vi "correction_data.vi"() -> ()   [LabVIEW 2020]
uses:
  CasaoManagerGeneralSpecifications.ctl
  General dimensions definition.ctl
  Point2D.ctl
  Point2Df.ctl
  Camera.lvclass
  WavefrontCorrector.lvclass
  CorrectionDataManager.lvclass
  Image.lvclass
  HasoEngine.lvclass
  InteractionMatrixToCommandMatrixParameters.ctl
  InteractionMatrixAcquisitionParameters.ctl
  HasoSlopes.lvclass
panel:
  in  "init_state_from_config_file":bool
  out "Camera Image (command 2)":u32[][](graph)
  in  "Start Acq":bool
  out "Singular values":dbl[](graph)
  in  "Correction data file name":string="Data\\data_correction_manager_example.aoc"
  in  "Exposure time (us)":i32=1000 min=1
  in  "number of images to sum":u32=1 min=1
  out "Camera Image (command 1)":u32[][](graph)
  in  "WavefrontCorrector Configuration file path":path
  out "error out":errorcluster
  out "Informations extracted \nfrom configuration files":T1 caption="Informations extracted from configuration files"
  in  "Haso configuration file path":path
  # "This example is Hardware-dependant, \nplease use your own Haso and corrector configuration file and acquisition system"
  # "Acquisition parameters"
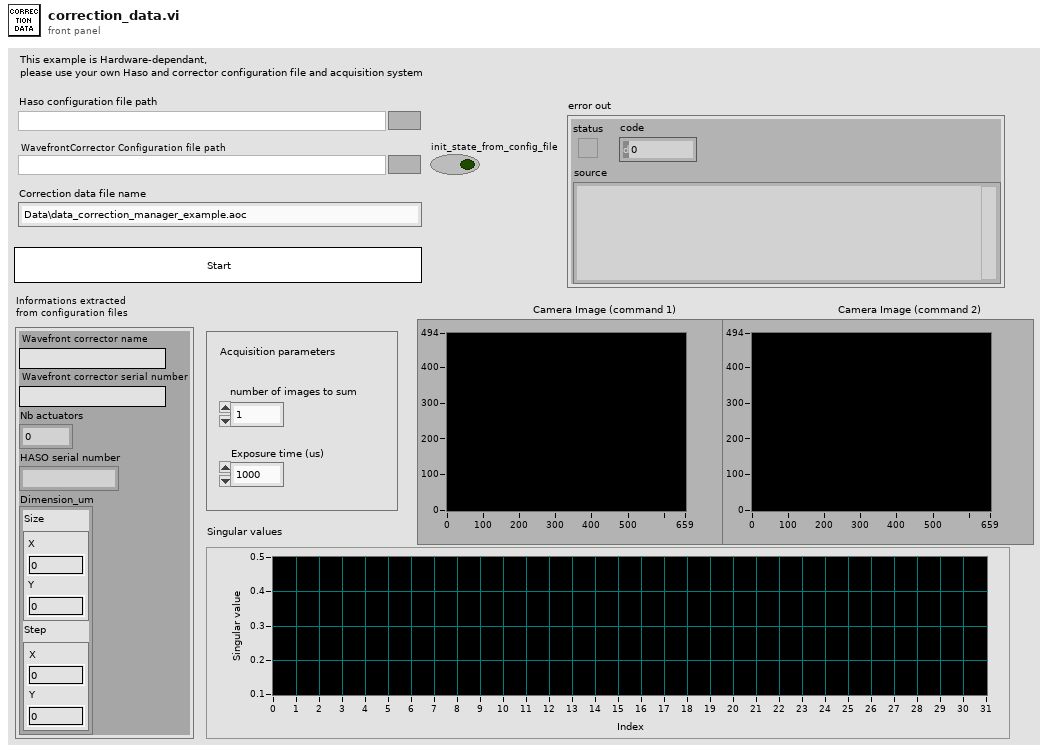
[diagram p1: front panel]
types:
  T1 = typedef "CasaoManagerGeneralSpecifications.ctl" = cluster{"Wavefront corrector name":string, "Wavefront corrector serial number":string, "Nb actuators":i32, "HASO serial number":string, "Dimension_um":T2}
  T2 = typedef "General dimensions definition.ctl" = cluster{"Size":T3, "Step":T4}
  T3 = typedef "Point2D.ctl" = cluster{"X":u32, "Y":u32}
  T4 = typedef "Point2Df.ctl" = cluster{"X":sgl, "Y":sgl}
  T5 = typedef "InteractionMatrixAcquisitionParameters.ctl" = cluster{"Push - Pull value":sgl}
  T6 = typedef "InteractionMatrixToCommandMatrixParameters.ctl" = cluster{"Number of kept modes":i32, "Tilt filtering":bool}
  T7 = typedef "Data alignment enum.ctl" = enum16{"8", "16", "32"}
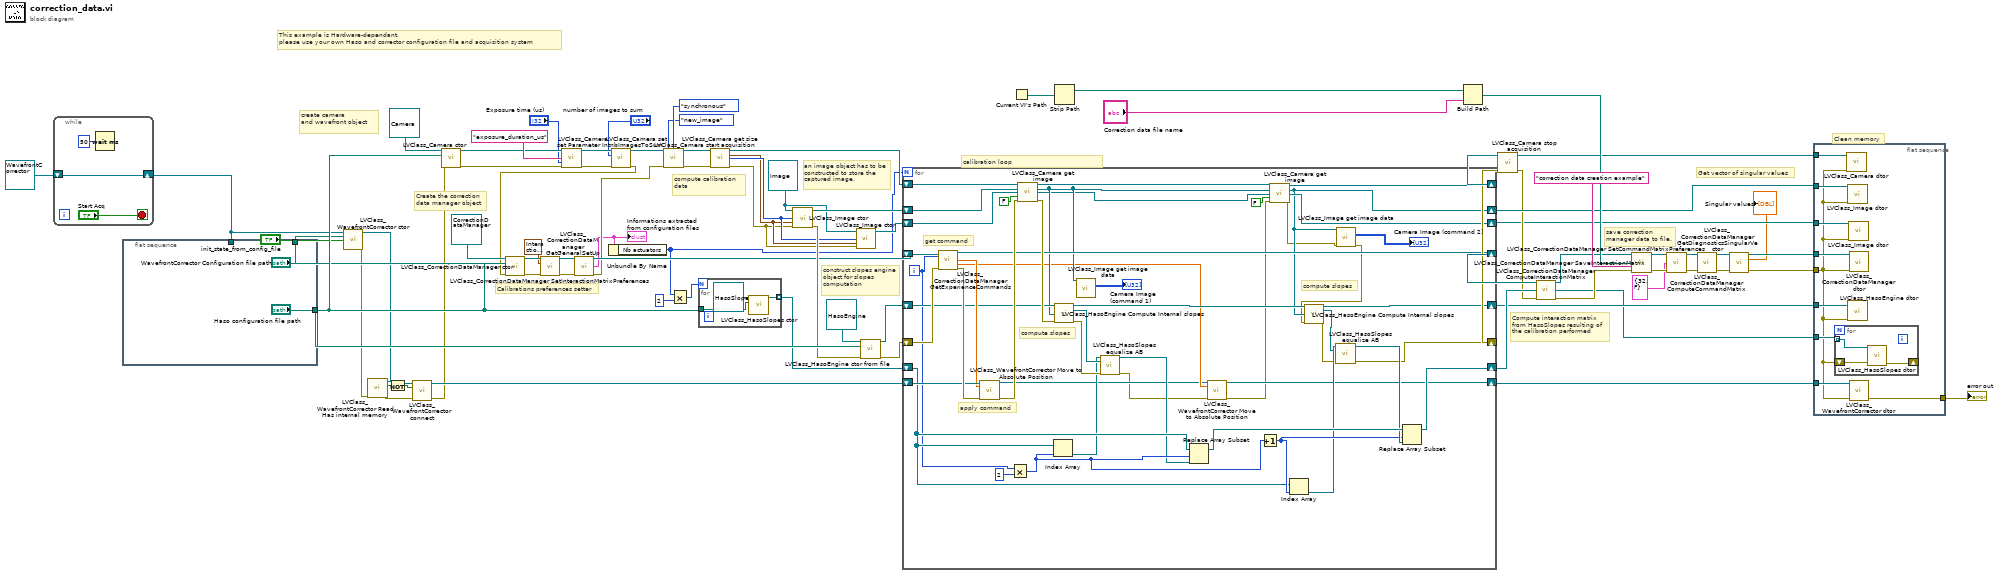
[diagram p0: block diagram]
diagram:
  w40 = refnum<class "Image.lvclass"> refnum ("Image in")
  # "Clean memory"
  # "Get vector of singular values"
  # "save correction\nmanager data to file."
  # "Compute interaction matrix\nfrom HasoSlopes resulting of\nthe calibration performed"
  # "calibration loop"
  # "construct slopes engine object for slopes computation"
  # "an image object has to be\nconstructed to store the\ncaptured image."
  # "compute calibration\ndata"
  # "Calibrations preferences setter"
  # "Create the correction\ndata manager object"
  # "create camera \nand wavefront object"
  # "This example is Hardware-dependant, \nplease use your own Haso and corrector configuration file and acquisition system"
  n1 = while {
    shift-right: [w82] -> w17
    shift-left: refnum<class "WavefrontCorrector.lvclass"> refnum ("WavefrontCorrector in") -> [w82]
    stop <- "Start Acq" stop-if-true
    n2 = Wait (ms)(milliseconds to wait=u32 50) -> ()  [unwired: 1 out]
  }
  n3 = flat-sequence {
    tunnel: ["Haso configuration file path"] -> w80
    tunnel: ["WavefrontCorrector Configuration file path"] -> w79
    tunnel: w17 -> [_]
    frame #0 {
    }
  }
  n4 = call "LVClass_WavefrontCorrector ctor.vi"("WavefrontCorrector (const)"=w17, "PathToWavefrontCorrectorSetupFile"=w79, "init_state_from_config_file"="init_state_from_config_file") -> ("WavefrontCorrector (new)"=w5:refnum<class "WavefrontCorrector.lvclass">, "error out"=w4:errorcluster)  [unwired: 11 in]
  n5 = call "LVClass_WavefrontCorrector Read Has internal memory.vi"("error in (no error)"=w4, "WavefrontCorrector in"=w5) -> ("error out"=w3:errorcluster, "Has internal memory ?"=w13:bool, "WavefrontCorrector out"=w14:refnum<class "WavefrontCorrector.lvclass">)  [unwired: 7 in]
  n6 = Not(x=w13) -> (.not. x?=w12:bool)
  n7 = call "LVClass_WavefrontCorrector connect.vi"("WavefrontCorrector in"=w14, "set_init_state_from_config_file"=w12, "error in (no error)"=w3) -> ("WavefrontCorrector out"=w15:refnum<class "WavefrontCorrector.lvclass">, "error out"=w2:errorcluster)  [unwired: 11 in]
  n8 = call "LVClass_Camera ctor.vi"("Camera (const)"=refnum<class "Camera.lvclass"> refnum ("Camera"), "Configuration file path"=w80, "error in (no error)"=w2) -> ("Camera (new)"=w28:refnum<class "Camera.lvclass">, "error out"=w22:errorcluster)  [unwired: 11 in]
  n9 = call "LVClass_Camera set Parameter Int.vi"("Camera in"=w28, "parameter_name"="exposure_duration_us", "value"="Exposure time (us)", "error in (no error)"=w22) -> ("Camera out"=w26:refnum<class "Camera.lvclass">, "error out"=w21:errorcluster)  [unwired: 10 in]
  n10 = call "LVClass_Camera set nbImagesToSum.vi"("Camera in"=w26, "nb_image"="number of images to sum", "error in (no error)"=w21) -> ("Camera out"=w25:refnum<class "Camera.lvclass">, "error out"=w20:errorcluster)  [unwired: 11 in]
  n11 = call "LVClass_CorrectionDataManager ctor.vi"("CorrectionDataManager (const)"=refnum<class "CorrectionDataManager.lvclass"> refnum ("CorrectionDataManager in"), "PathTohaso_config_file_path"=w80, "PathTowfc_config_file_path"=w79, "error in (no error)"=w20) -> ("CorrectionDataManager (new)"=w33:refnum<class "CorrectionDataManager.lvclass">, "error out"=w32:errorcluster)  [unwired: 10 in]
  n12 = call "LVClass_CorrectionDataManager SetInteractionMatrixPreferences.vi"("CorrectionDataManager in"=w33, "push_pull_value"=T5 {"Push - Pull value"=0.2}, "error in (no error)"=w32) -> ("CorrectionDataManager out"=w7:refnum<class "CorrectionDataManager.lvclass">, "error out"=w6:errorcluster)  [unwired: 11 in]
  n13 = call "LVClass_CorrectionDataManager GetGeneralSetUp.vi"("CorrectionDataManager in"=w7, "error in (no error)"=w6) -> ("CorrectionDataManager out"=w54:refnum<class "CorrectionDataManager.lvclass">, "general"=w11:T1, "error out"=w46:errorcluster)  [unwired: 11 in]
  "Informations extracted \nfrom configuration files" <- w11
  n14 = Unbundle By Name(w11) -> ("Nb actuators"=w10:i32)
  n15 = call "LVClass_Camera start acquisition.vi"("Camera in"=w25, "synchronisation_mode"=enum16{"synchronous", "asynchronous"}."synchronous", "acquisition_mode"=enum16{"last_image", "new_image"}."new_image", "error in (no error)"=w46) -> ("Camera out"=w47:refnum<class "Camera.lvclass">, "error out"=w45:errorcluster)  [unwired: 10 in]
  n16 = Multiply(x=w10, y=2) -> (x*y=w8:i32)
  n17 = for {
    N: w8 -> [_]
    tunnel: w80 -> [w88]
    tunnel: [w86] -> w49 mode=indexing
    n18 = call "LVClass_HasoSlopes ctor.vi"("HasoSlopes (const)"=refnum<class "HasoSlopes.lvclass"> refnum ("HasoSlopes in"), "Configuration file path"=w88) -> ("HasoSlopes (new)"=w86:refnum<class "HasoSlopes.lvclass">)  [unwired: 12 in, 1 out]
  }
  n19 = call "LVClass_Camera get size.vi"("Camera in"=w47, "error in (no error)"=w45) -> ("Camera out"=w69:refnum<class "Camera.lvclass">, "size"=w38:T3, "Number of bits"=w39:T7, "error out"=w37:errorcluster)  [unwired: 10 in]
  n20 = call "LVClass_Image ctor.vi"("Image (const)"=w40, "Data alignment"=w39, "Size"=w38, "error in (no error)"=w37) -> ("Image (new)"=w70:refnum<class "Image.lvclass">, "error out"=w75:errorcluster)  [unwired: 10 in]
  n21 = call "LVClass_Image ctor.vi"("Image (const)"=w40, "Data alignment"=w39, "Size"=w38, "error in (no error)"=w37) -> ("Image (new)"=w36:refnum<class "Image.lvclass">)  [unwired: 10 in, 1 out]
  n22 = call "LVClass_HasoEngine ctor from file.vi"("HasoEngine (const)"=refnum<class "HasoEngine.lvclass"> refnum ("HasoEngine in"), "Configuration file path"=w80, "error in (no error)"=w75) -> ("HasoEngine (new)"=w53:refnum<class "HasoEngine.lvclass">, "error out"=w74:errorcluster)  [unwired: 11 in]
  n23 = for {
    N: w10 -> [_]
    shift-right: [w94] -> w42
    shift-left: w74 -> [w135]
    shift-right: [w128] -> w61
    shift-left: w54 -> [w127]
    shift-right: [w108] -> w44
    shift-left: w69 -> [w131]
    shift-right: [w102] -> w51
    shift-left: w53 -> [w126]
    shift-right: [w91] -> w52
    shift-left: w70 -> [w121]
    shift-right: [w98] -> w50
    shift-left: w15 -> [w130]
    shift-right: [w105] -> w34
    shift-left: w36 -> [w123]
    shift-right: [w101] -> w68
    shift-left: w49 -> [w113]
    i -> [w93]
    # "compute slopes"
    # "compute slopes"
    # "apply command"
    # "get command"
    n24 = call "LVClass_CorrectionDataManager GetExperienceCommands.vi"("CorrectionDataManager in"=w127, "N° actuator"=w93, "error in (no error)"=w135) -> ("CorrectionDataManager out"=w128:refnum<class "CorrectionDataManager.lvclass">, "First DeltaCommand"=w129:sgl[], "Second DeltaCommand"=w100:sgl[], "error out"=w134:errorcluster)  [unwired: 9 in]
    n25 = call "LVClass_WavefrontCorrector Move to Absolute Position.vi"("WavefrontCorrector in"=w130, "Absolute Positions"=w129, "error in (no error)"=w134) -> ("WavefrontCorrector out"=w99:refnum<class "WavefrontCorrector.lvclass">, "error out"=w133:errorcluster)  [unwired: 11 in]
    n26 = Multiply(x=w93, y=2) -> (x*y=w116:i32)
    n27 = call "LVClass_Camera get image.vi"("Camera in"=w131, "Image"=w121, "Image RAW"=w123, "remove_background"=FALSE, "error in (no error)"=w133) -> ("Camera out"=w109:refnum<class "Camera.lvclass">, "Image (dup)"=w107:refnum<class "Image.lvclass">, "Image (dup) RAW"=w106:refnum<class "Image.lvclass">, "error out"=w132:errorcluster)  [unwired: 7 in]
    n28 = Index Array(array=w113, index=w116) -> (element=w112:refnum<class "HasoSlopes.lvclass">)
    n29 = call "LVClass_HasoEngine Compute Internal slopes.vi"("HasoEngine in"=w126, "Image.lvclass"=w107, "error in (no error)"=w132) -> ("HasoEngine out"=w103:refnum<class "HasoEngine.lvclass">, "HasoSlopes (dup)"=w124:refnum<class "HasoSlopes.lvclass">, "error out"=w125:errorcluster)  [unwired: 8 in, 2 out]
    n30 = call "LVClass_Image get image data.vi"("Image in"=w107) -> ("Image data out"=→"Camera Image (command 1)":u32[][])  [unwired: 12 in, 2 out]
    n31 = call "LVClass_HasoSlopes equalize AB.vi"("HasoSlopes dest in"=w112, "HasoSlopes source in"=w124, "error in (no error)"=w125) -> ("HasoSlopes dest out"=w111:refnum<class "HasoSlopes.lvclass">, "error out"=w96:errorcluster)  [unwired: 10 in, 1 out]
    n32 = Replace Array Subset(array=w113, new element=w111, index=w116) -> (w119:refnum<class "HasoSlopes.lvclass">[])
    n33 = call "LVClass_WavefrontCorrector Move to Absolute Position.vi"("WavefrontCorrector in"=w99, "Absolute Positions"=w100, "error in (no error)"=w96) -> ("WavefrontCorrector out"=w98:refnum<class "WavefrontCorrector.lvclass">, "error out"=w97:errorcluster)  [unwired: 11 in]
    n34 = Increment(x=w116) -> (x+1=w115:i32)
    n35 = call "LVClass_Camera get image.vi"("Camera in"=w109, "Image"=w107, "Image RAW"=w106, "remove_background"=FALSE, "error in (no error)"=w97) -> ("Camera out"=w108:refnum<class "Camera.lvclass">, "Image (dup)"=w91:refnum<class "Image.lvclass">, "Image (dup) RAW"=w105:refnum<class "Image.lvclass">, "error out"=w90:errorcluster)  [unwired: 7 in]
    n36 = Index Array(array=w113, index=w115) -> (element=w114:refnum<class "HasoSlopes.lvclass">)
    n37 = call "LVClass_Image get image data.vi"("Image in"=w91, "error in (no error)"=w90) -> ("Image data out"=→"Camera Image (command 2)":u32[][], "error out"=w89:errorcluster)  [unwired: 11 in, 1 out]
    n38 = call "LVClass_HasoEngine Compute Internal slopes.vi"("HasoEngine in"=w103, "Image.lvclass"=w91, "error in (no error)"=w89) -> ("HasoEngine out"=w102:refnum<class "HasoEngine.lvclass">, "HasoSlopes (dup)"=w104:refnum<class "HasoSlopes.lvclass">, "error out"=w95:errorcluster)  [unwired: 8 in, 2 out]
    n39 = call "LVClass_HasoSlopes equalize AB.vi"("HasoSlopes dest in"=w114, "HasoSlopes source in"=w104, "error in (no error)"=w95) -> ("HasoSlopes dest out"=w118:refnum<class "HasoSlopes.lvclass">, "error out"=w94:errorcluster)  [unwired: 10 in, 1 out]
    n40 = Replace Array Subset(array=w119, new element=w118, index=w115) -> (w101:refnum<class "HasoSlopes.lvclass">[])
  }
  n41 = Current VI's Path() -> (path=w18:path)
  n42 = Strip Path(path=w18) -> (stripped path=w67:path)  [unwired: 1 out]
  n43 = Build Path(base path=w67, name or relative path="Correction data file name") -> (appended path=w65:path)
  n44 = call "LVClass_Camera stop acquisition.vi"("Camera in"=w44, "error in (no error)"=w42) -> ("Camera out"=w43:refnum<class "Camera.lvclass">, "error out"=w41:errorcluster)  [unwired: 12 in]
  n45 = call "LVClass_CorrectionDataManager ComputeInteractionMatrix.vi"("CorrectionDataManager in"=w61, "HasoSlopes array"=w68, "error in (no error)"=w41) -> ("CorrectionDataManager out"=w62:refnum<class "CorrectionDataManager.lvclass">, "HasoSlopes array 2"=w48:refnum<class "HasoSlopes.lvclass">[], "error out"=w73:errorcluster)  [unwired: 10 in]
  n46 = call "LVClass_CorrectionDataManager SaveInteractrionMatrix.vi"("CorrectionDataManager in"=w62, "Interaction Matrix file path"=w65, "comment"="correction data creation example", "error in (no error)"=w73) -> ("CorrectionDataManager out"=w60:refnum<class "CorrectionDataManager.lvclass">, "error out"=w72:errorcluster)  [unwired: 10 in]
  n47 = call "LVClass_CorrectionDataManager SetCommandMatrixPreferences.vi"("CorrectionDataManager in"=w60, "Prefs"=T6 {"Number of kept modes"=32, "Tilt filtering"=FALSE}, "error in (no error)"=w72) -> ("CorrectionDataManager out"=w59:refnum<class "CorrectionDataManager.lvclass">, "error out"=w56:errorcluster)  [unwired: 11 in]
  n48 = call "LVClass_CorrectionDataManager ComputeCommandMatrix.vi"("CorrectionDataManager in"=w59, "error in (no error)"=w56) -> ("CorrectionDataManager out"=w58:refnum<class "CorrectionDataManager.lvclass">, "error out"=w57:errorcluster)  [unwired: 12 in]
  n49 = call "LVClass_CorrectionDataManager GetDiagnosticsSingularVector.vi"("CorrectionDataManager in"=w58, "error in (no error)"=w57) -> ("CorrectionDataManager out"=w55:refnum<class "CorrectionDataManager.lvclass">, "ArrayOfSingularValues"=→"Singular values":dbl[], "error out"=w35:errorcluster)  [unwired: 11 in]
  n50 = flat-sequence {
    tunnel: w55 -> [w144]
    tunnel: w52 -> [w143]
    tunnel: w51 -> [w142]
    tunnel: w50 -> [w141]
    tunnel: w48 -> [w140]
    tunnel: w43 -> [w139]
    tunnel: w35 -> [w136]
    tunnel: w34 -> [w138]
    tunnel: [w137] -> w78
    frame #0 {
      n51 = for {
        tunnel: w140 -> [w147] mode=indexing
        shift-right: [w145] -> _
        shift-left: w136 -> [w146]
        n52 = call "LVClass_HasoSlopes dtor.vi"("HasoSlopes in"=w147, "error in (no error)"=w146) -> ("error out"=w145:errorcluster)  [unwired: 12 in, 1 out]
      }
      n53 = call "LVClass_Camera dtor.vi"("Camera in"=w139, "error in (no error)"=w136) -> ()  [unwired: 12 in, 2 out]
      n54 = call "LVClass_Image dtor.vi"("Image in"=w143, "error in (no error)"=w136) -> ()  [unwired: 12 in, 2 out]
      n55 = call "LVClass_HasoEngine dtor.vi"("HasoEngine in"=w142, "error in (no error)"=w136) -> ()  [unwired: 12 in, 2 out]
      n56 = call "LVClass_Image dtor.vi"("Image in"=w138, "error in (no error)"=w136) -> ()  [unwired: 12 in, 2 out]
      n57 = call "LVClass_CorrectionDataManager dtor.vi"("CorrectionDataManager in"=w144, "error in (no error)"=w136) -> ()  [unwired: 12 in, 2 out]
      n58 = call "LVClass_WavefrontCorrector dtor.vi"("WavefrontCorrector in"=w141, "error in (no error)"=w136) -> ("error out"=w137:errorcluster)  [unwired: 12 in, 1 out]
    }
  }
  "error out" <- w78
